vi "To work on 1.vi"(1 "error in (no error)":errorcluster, 2 "Объекты":T1={"Ускоренно/Реально"=TRUE, "Станок 1"={"Время на обработку (с)"=40, "Шанс брака (%)"=4.0}, "Станок 2"={"Время на обработку (с)"=60, "Шанс брака (%)"=8.0}, "Кол-во деталей"=500, "Задержки на перемещение"={"Время загрузки\n первого станка (с)"=5, "Время загрузки\n второго станка (с) "=6, "Время до урны (с)"=3, "Время до коробки (с)"=2, "Время между станками (с)"=3}, "Повторная \nобработка\n на станке:"=TRUE}) -> (0 "error out":errorcluster)   [LabVIEW 2020]
uses:
  Var/Global 1.vi
panel:
  # "1"
  # "2"
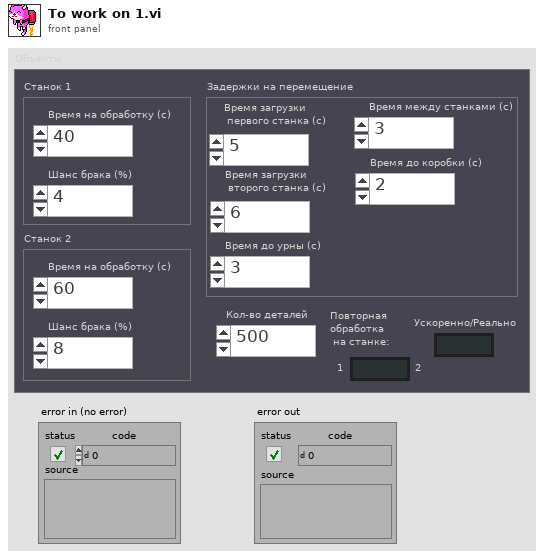
[diagram p1: front panel]
types:
  T1 = cluster{"Ускоренно/Реально":bool, "Станок 1":cluster{"Время на обработку (с)":i32, "Шанс брака (%)":dbl}, "Станок 2":cluster{"Время на обработку (с)":i32, "Шанс брака (%)":dbl}, "Кол-во деталей":i32, "Задержки на перемещение":cluster{"Время загрузки\n первого станка (с)":i32, "Время загрузки\n второго станка (с) ":i32, "Время до урны (с)":i32, "Время до коробки (с)":i32, "Время между станками (с)":i32}, "Повторная \nобработка\n на станке:":bool}
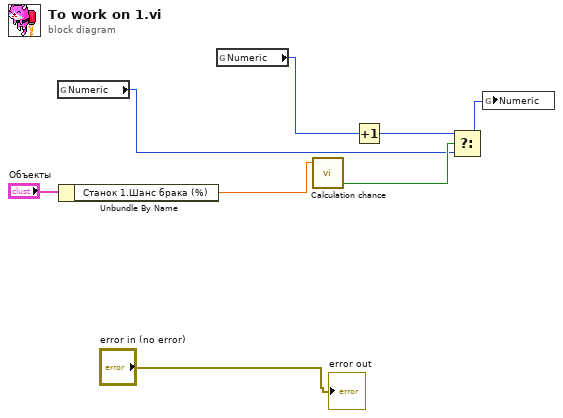
[diagram p0: block diagram]
diagram:
  n1 = global read "Global 1.vi" "Numeric"() -> (w5:i32)
  n2 = Unbundle By Name("Объекты") -> ("Станок 1.Шанс брака (%)"=w7:dbl)
  n3 = global read "Global 1.vi" "Numeric"() -> (w4:i32)
  n4 = call "Calculation chance.vi"("Defective (%)"=w7) -> ("x > y?"=w6:bool)  [unwired: 1 in]
  n5 = Increment(x=w4) -> (x+1=w3:i32)
  n6 = Select(t=w3, s=w6, f=w5) -> (s? t:f=w2:i32)
  n7 = global write "Global 1.vi" "Numeric"(w2) -> ()
  "error out" <- "error in (no error)"
